vi "ProyectoFinalVI.vi"() -> ()   [LabVIEW 2025]
uses:
  <vilib>/httpClient/PUTBuffer.vi
  <vilib>/httpClient/LabVIEWHTTPClient.lvlib
panel:
  in  "Tab Control":T1(tab)
  out "Planta":dbl(knob)
  in  "OK Button":bool
  in  "Set-Point":dbl(knob) scale=0.0..360.0
  in  "KP":dbl
  out "error PUT":errorcluster
  out "headers PUT":string
  out "body PUT":string
  in  "KI":dbl
  in  "KD":dbl
  in  "Dt":dbl
  out "SET-POINT":dbl
  out "KP":dbl
  out "KI":dbl
  out "KD":dbl
  out "Dt":dbl
  out "POS":dbl
  out "error GET":errorcluster
  out "headers GET":string
  out "body GET":string
  out "Boolean 2":bool
  out "Boolean":bool
  out "Secuencia":string
  out "Aceptar":bool
  out "error GET 2":errorcluster
  out "body GET 2":string
  out "headers GET 2":string
  out "error PUT 2":errorcluster
  out "body PUT 2":string
  out "headers PUT 2":string
  in  "Secuencia 2":string
  in  "Aceptar 2":bool
  in  "OK Button 2":bool
  out "Tank":dbl(slide) scale=0.0..100.0
  out "KP 2":dbl
  out "KI 2":dbl
  out "RPM":dbl
  out "error GET 3":errorcluster
  out "body GET 3":string
  out "headers GET 3":string
  out "error PUT 3":errorcluster
  out "body PUT 3":string
  out "headers PUT 3":string
  in  "OK Button 3":bool
  in  "KP 3":dbl
  in  "KI 3":dbl
  in  "RPM 2":dbl
  out "Thermometer":dbl(slide) scale=0.0..100.0
  out "K":dbl
  out "Ki":dbl
  out "Kd":dbl
  out "SetPoint":dbl
  out "Temp":dbl
  out "error GET 4":errorcluster
  out "body GET 4":string
  out "headers GET 4":string
  out "error PUT 4":errorcluster
  out "body PUT 4":string
  out "headers PUT 4":string
  in  "OK Button 4":bool
  in  "K 2":dbl
  in  "Ki 2":dbl
  in  "Kd 2":dbl
  in  "SetPoint 2":dbl
  in  "Temp 2":dbl
  out "KP 4":dbl
  out "KI 4":dbl
  out "RPM 3":dbl
  in  "KP 5":dbl
  in  "KI 5":dbl
  in  "RPM 4":dbl
  in  "OK Button 5":bool
  out "error GET 5":errorcluster
  out "body GET 5":string
  out "headers GET 5":string
  out "error PUT 5":errorcluster
  out "body PUT 5":string
  out "headers PUT 5":string
  out "K 3":dbl
  out "Ki 3":dbl
  out "Kd 3":dbl
  out "sp":dbl
  in  "K 4":dbl
  in  "Ki 4":dbl
  in  "Kd 4":dbl
  in  "sp 2":dbl
  in  "OK Button 6":bool
  out "error GET 6":errorcluster
  out "body GET 6":string
  out "headers GET 6":string
  out "error PUT 6":errorcluster
  out "body PUT 6":string
  out "headers PUT 6":string
  out "error GET 7":errorcluster
  out "body GET 7":string
  out "headers GET 7":string
  out "error PUT 7":errorcluster
  out "body PUT 7":string
  out "headers PUT 7":string
  out "KP 6":dbl
  out "KI 6":dbl
  out "RPM 5":dbl
  in  "KP 7":dbl
  in  "KI 7":dbl
  in  "RPM 6":dbl
  in  "OK Button 7":bool
  in  "stop":bool
  # "Instituto Politécnico Nacional"
  # "Unidad Profesional Interdisciplinaria de Ingeniería Campus Zacatecas"
  # "Instrumentación Virtual Aplicada"
  # "Current Data"
  # "Send Data"
  # "Current Data"
  # "Send Data"
  # "Current Data"
  # "Send Data"
  # "Current Data"
  # "Send Data"
  # "Current Data"
  # "Send Data"
  # "Current Data"
  # "Send Data"
  # "Current Data"
  # "Current Data"
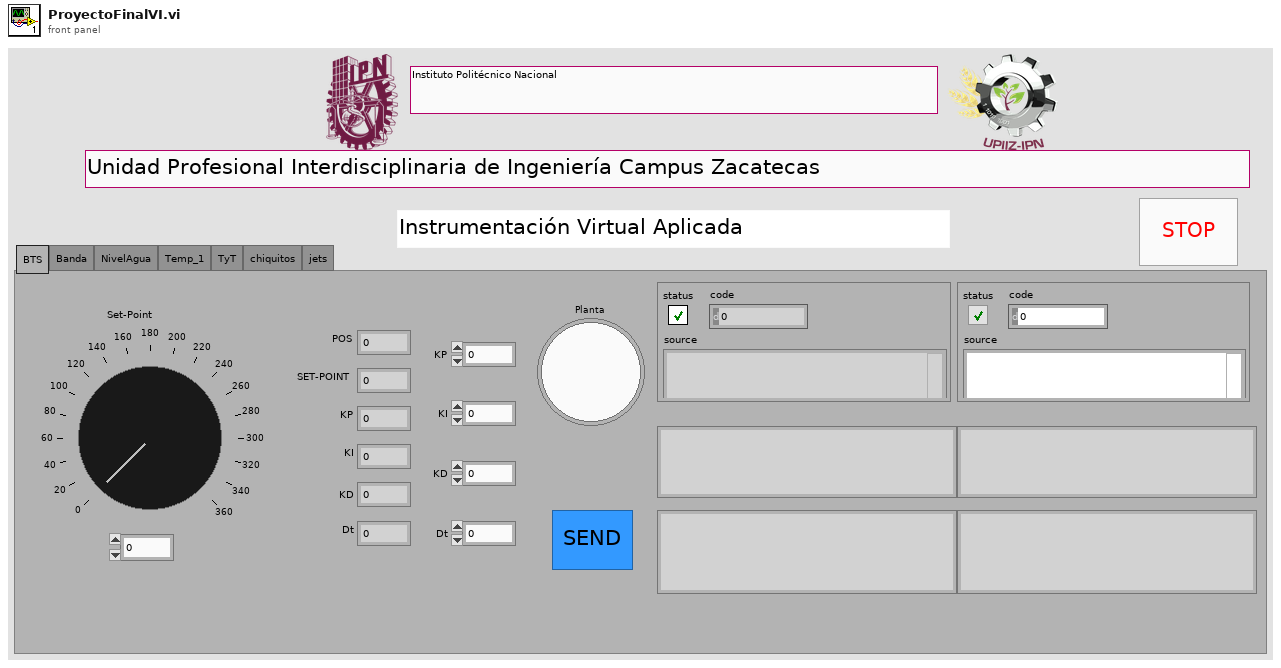
[diagram p1: front panel]
types:
  T1 = enum32{"BTS", "Banda", "NivelAgua", "Temp_1", "TyT", "chiquitos", "jets"}
  T2 = cluster{"Sensor":dbl, "Set-Point":dbl, "kp":dbl, "ki":dbl, "kd":dbl, "dt":dbl}
  T3 = cluster{"Set-Point":dbl, "kp":dbl, "ki":dbl, "kd":dbl, "dt":dbl, "Sensor":dbl}
  T4 = cluster{"K":dbl, "Ki":dbl, "Kd":dbl, "SetPoint":dbl, "Temp":dbl}
  T5 = cluster{"Kd":dbl, "Ki":dbl, "SetPoint":dbl, "Temp":dbl, "K":dbl}
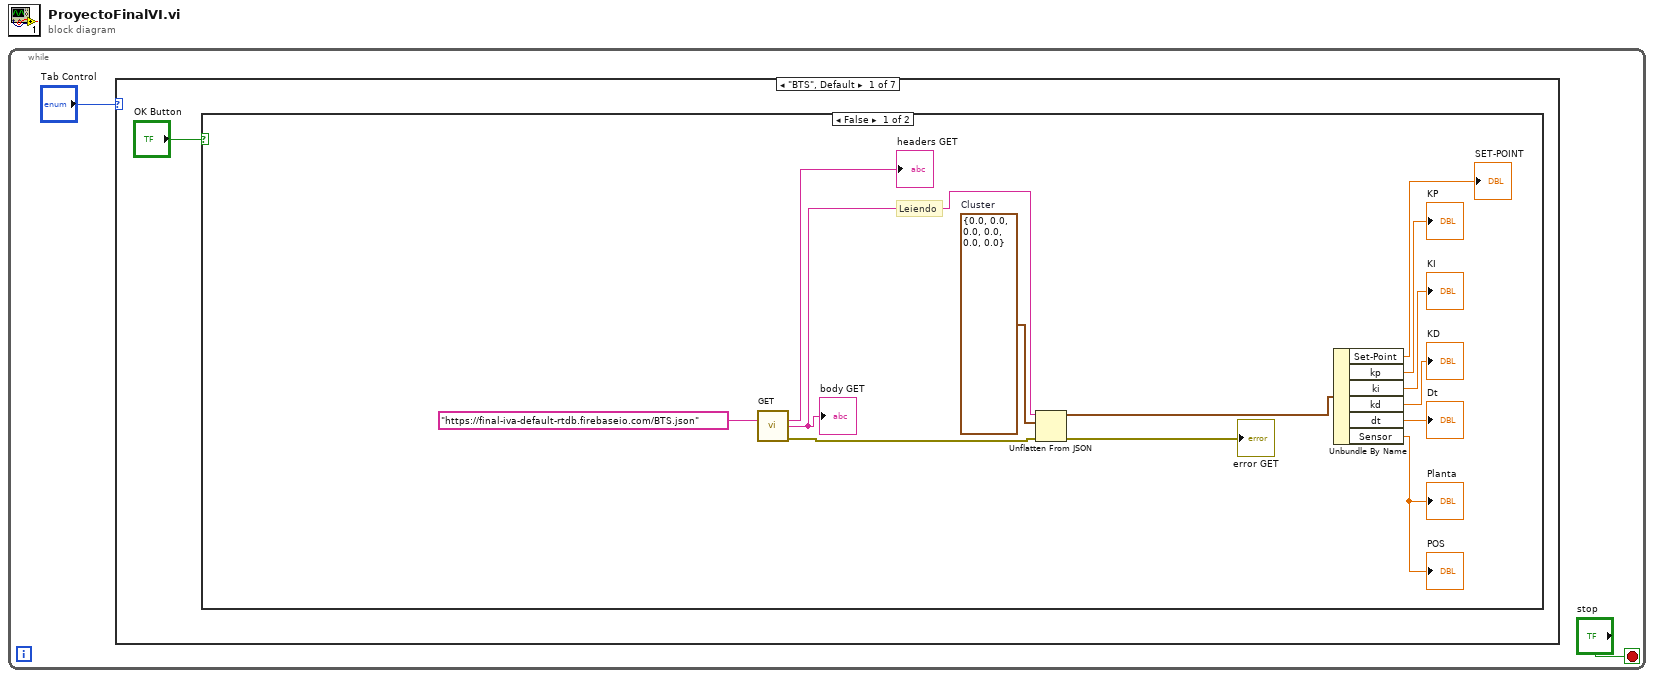
[diagram p0: block diagram]
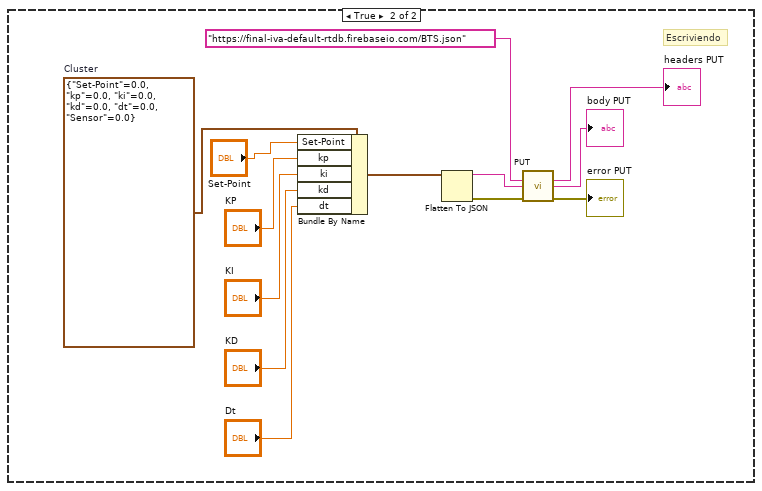
[diagram p2: hidden frame]
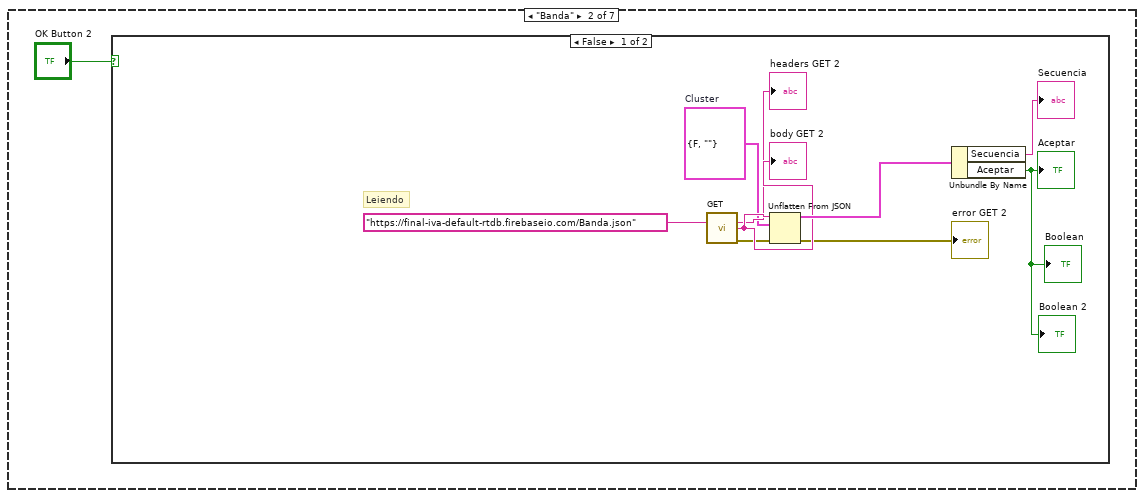
[diagram p3: hidden frame]
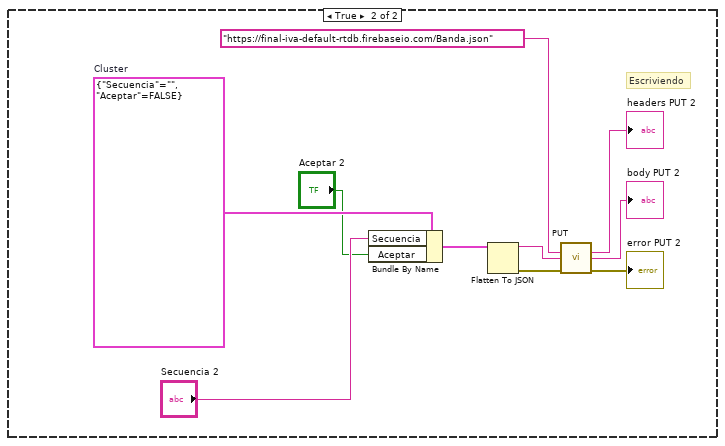
[diagram p4: hidden frame]
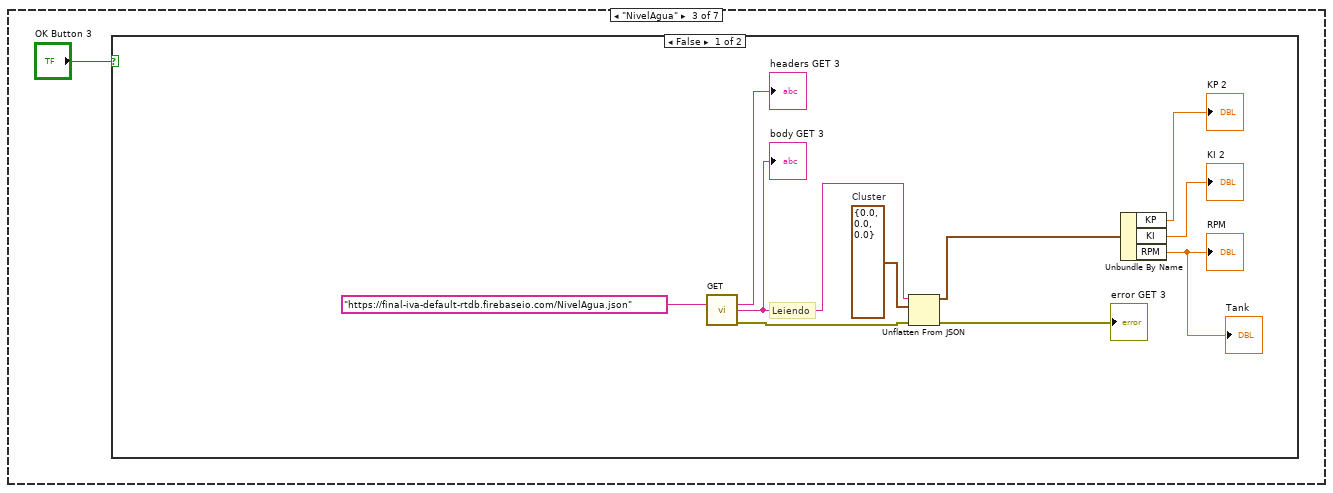
[diagram p5: hidden frame]
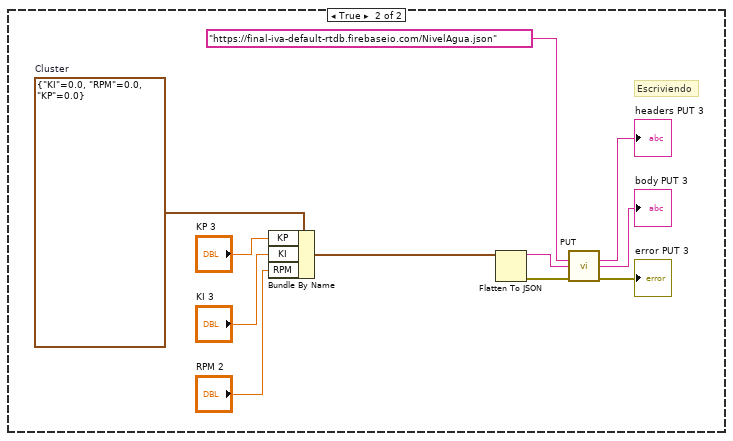
[diagram p6: hidden frame]
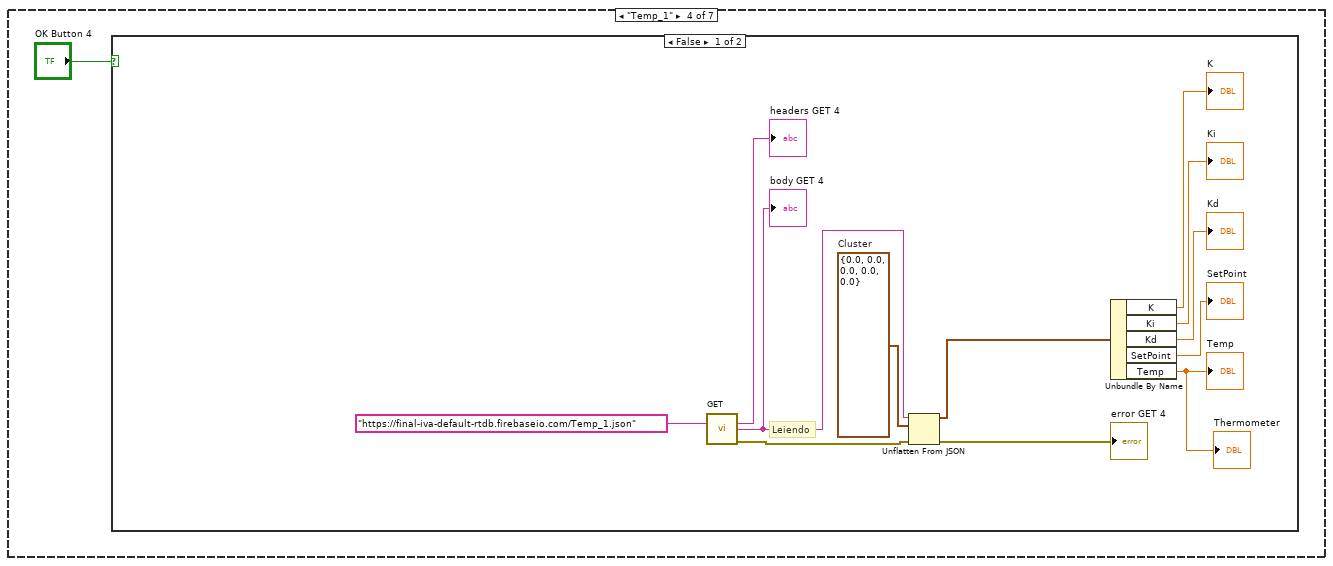
[diagram p7: hidden frame]
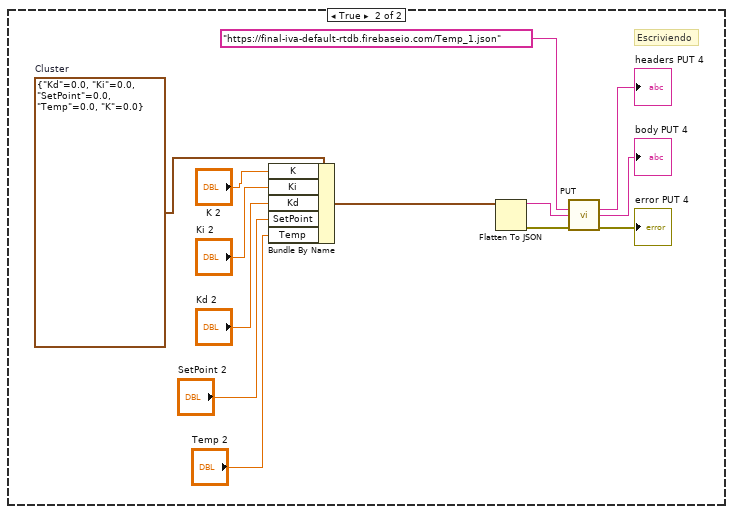
[diagram p8: hidden frame]
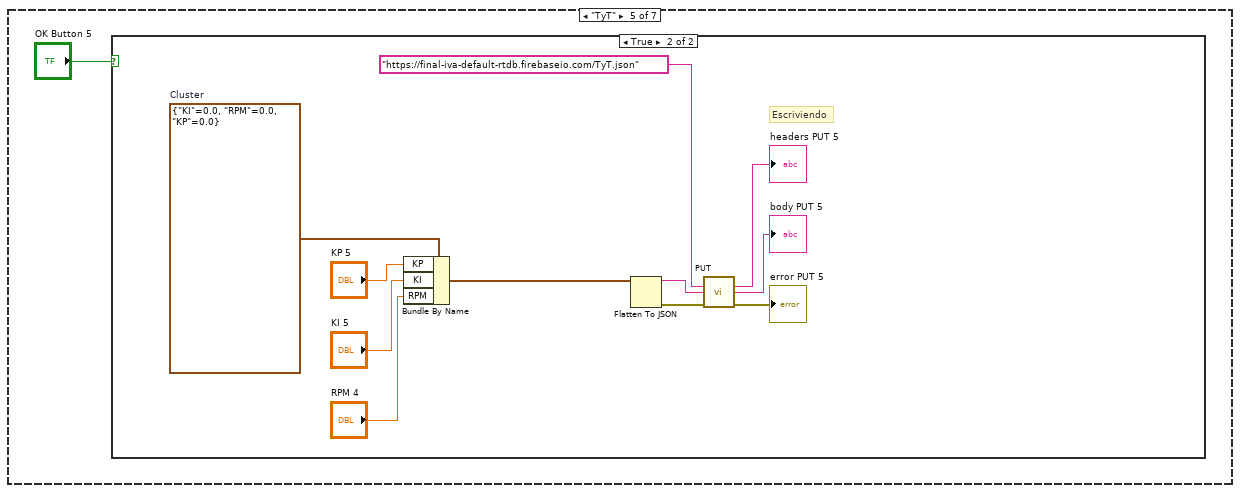
[diagram p9: hidden frame]
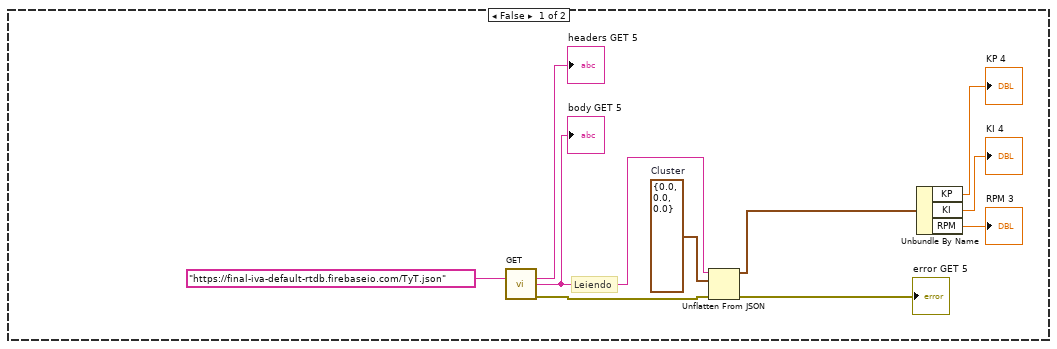
[diagram p10: hidden frame]
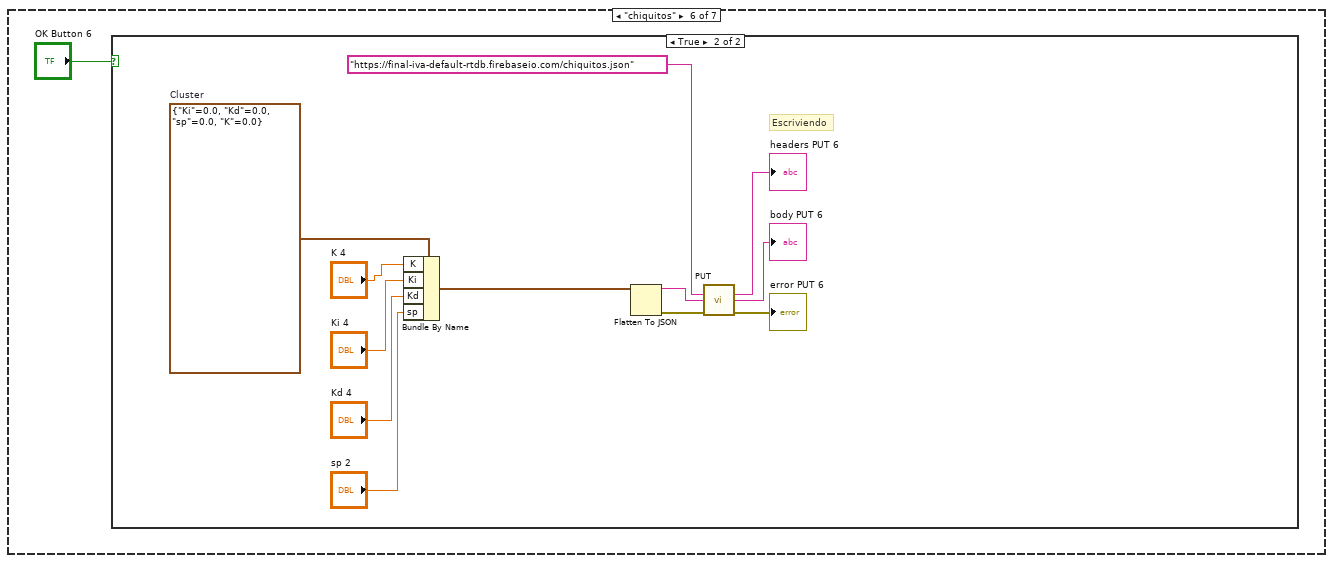
[diagram p11: hidden frame]
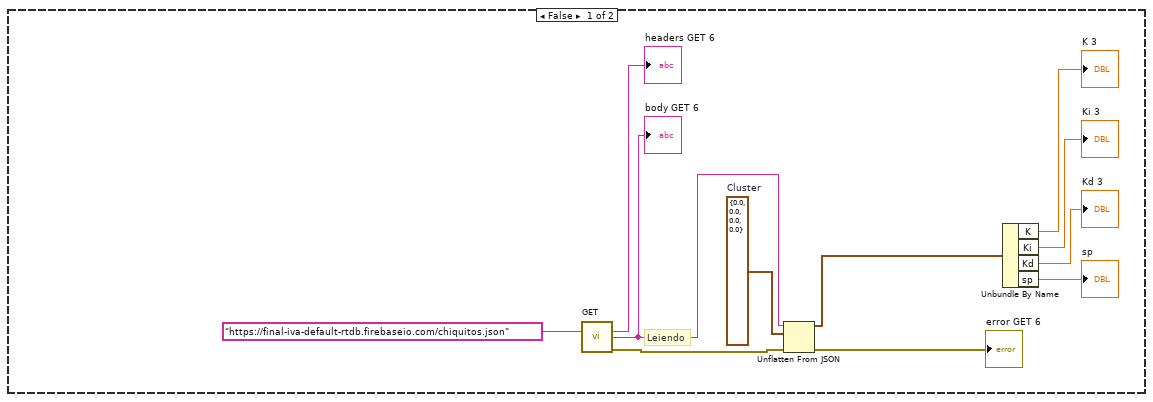
[diagram p12: hidden frame]
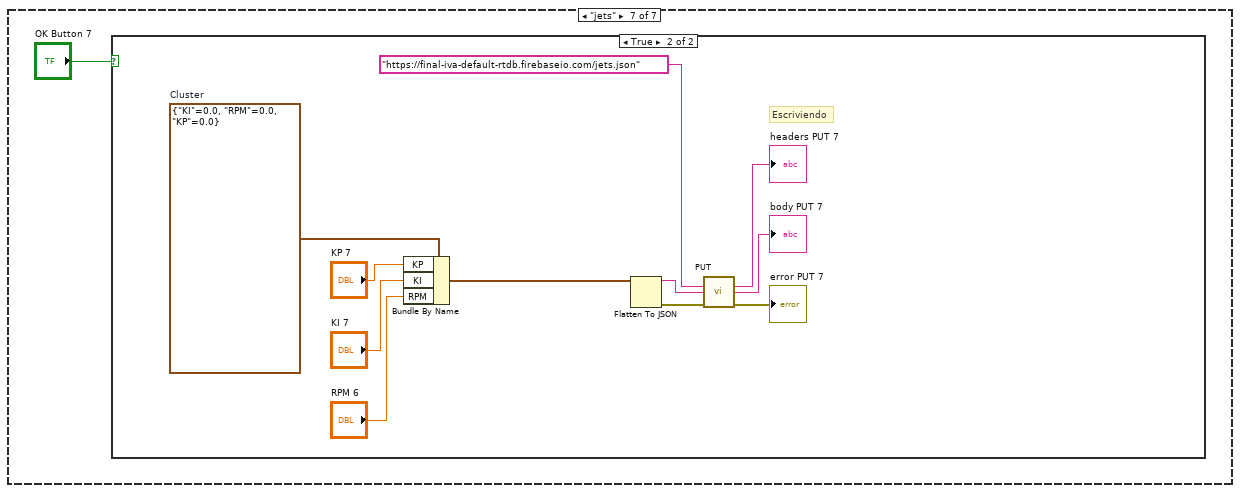
[diagram p13: hidden frame]
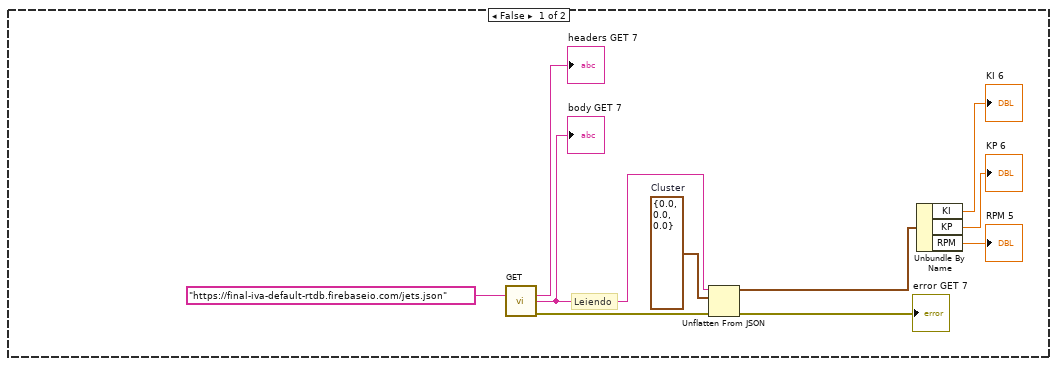
[diagram p14: hidden frame]
diagram:
  n1 = while {
    stop <- "stop" stop-if-true
    n2 = case shown="\"BTS\", Default" "Tab Control" {
      frame "BTS", Default {
        n3 = case shown="False" "OK Button" {
          frame False {
            w10 = T2 {"Sensor"=0.0, "Set-Point"=0.0, "kp"=0.0, "ki"=0.0, "kd"=0.0, "dt"=0.0}  # Cluster
            # "Leiendo"
            n4 = call <vilib>:"GET.vi"("url"="https://final-iva-default-rtdb.firebaseio.com/BTS.json") -> ("headers"=→"headers GET":string, "body"=w15:string, "error out"=w12:errorcluster)  [unwired: 11 in, 1 out]
            "body GET" <- w15
            n5 = Unflatten From JSON(JSON string=w15, type and defaults=w10, error in (no error)=w12) -> (value=w16:T2, error out=→"error GET":errorcluster)  [unwired: 4 in]
            n6 = Unbundle By Name(w16) -> ("Set-Point"=→"SET-POINT":dbl, "kp"=→"KP":dbl, "ki"=→"KI":dbl, "kd"=→"KD":dbl, "dt"=→"Dt":dbl, "Sensor"=→"POS" →"Planta":dbl)
          }
          frame True {
            w23 = T3 {"Set-Point"=0.0, "kp"=0.0, "ki"=0.0, "kd"=0.0, "dt"=0.0, "Sensor"=0.0}  # Cluster
            # "Escriviendo"
            n7 = Bundle By Name "Bundle By Name"(cluster=w23, "Set-Point"="Set-Point", "kp"="KP", "ki"="KI", "kd"="KD", "dt"="Dt") -> (w29:T3)
            n8 = Flatten To JSON(anything=w29) -> (JSON string=w26:string, 11:w22:errorcluster)  [unwired: 2 in]
            n9 = call-poly <vilib>:"PUT.vi"("url"="https://final-iva-default-rtdb.firebaseio.com/BTS.json", "buffer"=w26, "error in (no error)"=w22) -> ("headers"=→"headers PUT":string, "body"=→"body PUT":string, "error out"=→"error PUT":errorcluster)  [unwired: 9 in, 1 out]
          }
        }
      }
      frame "Banda" {
        n10 = case shown="False" "OK Button 2" {
          frame False {
            w33 = cluster{"Aceptar":bool, "Secuencia":string} {"Aceptar"=FALSE, "Secuencia"=""}  # Cluster
            # "Leiendo"
            n11 = call <vilib>:"GET.vi"("url"="https://final-iva-default-rtdb.firebaseio.com/Banda.json") -> ("headers"=→"headers GET 2":string, "body"=w38:string, "error out"=w35:errorcluster)  [unwired: 11 in, 1 out]
            "body GET 2" <- w38
            n12 = Unflatten From JSON(JSON string=w38, type and defaults=w33, error in (no error)=w35) -> (value=w39:cluster{"Aceptar":bool, "Secuencia":string}, error out=→"error GET 2":errorcluster)  [unwired: 4 in]
            n13 = Unbundle By Name(w39) -> ("Secuencia"=→"Secuencia":string, "Aceptar"=→"Aceptar" →"Boolean" →"Boolean 2":bool)
          }
          frame True {
            w43 = cluster{"Secuencia":string, "Aceptar":bool} {"Secuencia"="", "Aceptar"=FALSE}  # Cluster
            # "Escriviendo"
            n14 = Bundle By Name "Bundle By Name"(cluster=w43, "Secuencia"="Secuencia 2", "Aceptar"="Aceptar 2") -> (w49:cluster{"Secuencia":string, "Aceptar":bool})
            n15 = Flatten To JSON(anything=w49) -> (JSON string=w46:string, 11:w42:errorcluster)  [unwired: 2 in]
            n16 = call-poly <vilib>:"PUT.vi"("url"="https://final-iva-default-rtdb.firebaseio.com/Banda.json", "buffer"=w46, "error in (no error)"=w42) -> ("headers"=→"headers PUT 2":string, "body"=→"body PUT 2":string, "error out"=→"error PUT 2":errorcluster)  [unwired: 9 in, 1 out]
          }
        }
      }
      frame "NivelAgua" {
        n17 = case shown="False" "OK Button 3" {
          frame False {
            w54 = cluster{"KP":dbl, "KI":dbl, "RPM":dbl} {"KP"=0.0, "KI"=0.0, "RPM"=0.0}  # Cluster
            # "Leiendo"
            n18 = call <vilib>:"GET.vi"("url"="https://final-iva-default-rtdb.firebaseio.com/NivelAgua.json") -> ("headers"=→"headers GET 3":string, "body"=w59:string, "error out"=w56:errorcluster)  [unwired: 11 in, 1 out]
            "body GET 3" <- w59
            n19 = Unflatten From JSON(JSON string=w59, type and defaults=w54, error in (no error)=w56) -> (value=w60:cluster{"KP":dbl, "KI":dbl, "RPM":dbl}, error out=→"error GET 3":errorcluster)  [unwired: 4 in]
            n20 = Unbundle By Name(w60) -> ("KP"=→"KP 2":dbl, "KI"=→"KI 2":dbl, "RPM"=→"RPM" →"Tank":dbl)
          }
          frame True {
            w65 = cluster{"KI":dbl, "RPM":dbl, "KP":dbl} {"KI"=0.0, "RPM"=0.0, "KP"=0.0}  # Cluster
            # "Escriviendo"
            n21 = Bundle By Name "Bundle By Name"(cluster=w65, "KP"="KP 3", "KI"="KI 3", "RPM"="RPM 2") -> (w71:cluster{"KI":dbl, "RPM":dbl, "KP":dbl})
            n22 = Flatten To JSON(anything=w71) -> (JSON string=w68:string, 11:w64:errorcluster)  [unwired: 2 in]
            n23 = call-poly <vilib>:"PUT.vi"("url"="https://final-iva-default-rtdb.firebaseio.com/NivelAgua.json", "buffer"=w68, "error in (no error)"=w64) -> ("headers"=→"headers PUT 3":string, "body"=→"body PUT 3":string, "error out"=→"error PUT 3":errorcluster)  [unwired: 9 in, 1 out]
          }
        }
      }
      frame "Temp_1" {
        n24 = case shown="False" "OK Button 4" {
          frame False {
            w78 = T4 {"K"=0.0, "Ki"=0.0, "Kd"=0.0, "SetPoint"=0.0, "Temp"=0.0}  # Cluster
            # "Leiendo"
            n25 = call <vilib>:"GET.vi"("url"="https://final-iva-default-rtdb.firebaseio.com/Temp_1.json") -> ("headers"=→"headers GET 4":string, "body"=w83:string, "error out"=w80:errorcluster)  [unwired: 11 in, 1 out]
            "body GET 4" <- w83
            n26 = Unflatten From JSON(JSON string=w83, type and defaults=w78, error in (no error)=w80) -> (value=w84:T4, error out=→"error GET 4":errorcluster)  [unwired: 4 in]
            n27 = Unbundle By Name(w84) -> ("K"=→"K":dbl, "Ki"=→"Ki":dbl, "Kd"=→"Kd":dbl, "SetPoint"=→"SetPoint":dbl, "Temp"=→"Temp" →"Thermometer":dbl)
          }
          frame True {
            w91 = T5 {"Kd"=0.0, "Ki"=0.0, "SetPoint"=0.0, "Temp"=0.0, "K"=0.0}  # Cluster
            # "Escriviendo"
            n28 = Bundle By Name "Bundle By Name"(cluster=w91, "K"="K 2", "Ki"="Ki 2", "Kd"="Kd 2", "SetPoint"="SetPoint 2", "Temp"="Temp 2") -> (w97:T5)
            n29 = Flatten To JSON(anything=w97) -> (JSON string=w94:string, 11:w90:errorcluster)  [unwired: 2 in]
            n30 = call-poly <vilib>:"PUT.vi"("url"="https://final-iva-default-rtdb.firebaseio.com/Temp_1.json", "buffer"=w94, "error in (no error)"=w90) -> ("headers"=→"headers PUT 4":string, "body"=→"body PUT 4":string, "error out"=→"error PUT 4":errorcluster)  [unwired: 9 in, 1 out]
          }
        }
      }
      frame "TyT" {
        n31 = case shown="True" "OK Button 5" {
          frame False {
            w102 = cluster{"KP":dbl, "KI":dbl, "RPM":dbl} {"KP"=0.0, "KI"=0.0, "RPM"=0.0}  # Cluster
            # "Leiendo"
            n32 = call <vilib>:"GET.vi"("url"="https://final-iva-default-rtdb.firebaseio.com/TyT.json") -> ("headers"=→"headers GET 5":string, "body"=w107:string, "error out"=w104:errorcluster)  [unwired: 11 in, 1 out]
            "body GET 5" <- w107
            n33 = Unflatten From JSON(JSON string=w107, type and defaults=w102, error in (no error)=w104) -> (value=w108:cluster{"KP":dbl, "KI":dbl, "RPM":dbl}, error out=→"error GET 5":errorcluster)  [unwired: 4 in]
            n34 = Unbundle By Name(w108) -> ("KP"=→"KP 4":dbl, "KI"=→"KI 4":dbl, "RPM"=→"RPM 3":dbl)
          }
          frame True {
            w113 = cluster{"KI":dbl, "RPM":dbl, "KP":dbl} {"KI"=0.0, "RPM"=0.0, "KP"=0.0}  # Cluster
            # "Escriviendo"
            n35 = Bundle By Name "Bundle By Name"(cluster=w113, "KP"="KP 5", "KI"="KI 5", "RPM"="RPM 4") -> (w119:cluster{"KI":dbl, "RPM":dbl, "KP":dbl})
            n36 = Flatten To JSON(anything=w119) -> (JSON string=w116:string, 11:w112:errorcluster)  [unwired: 2 in]
            n37 = call-poly <vilib>:"PUT.vi"("url"="https://final-iva-default-rtdb.firebaseio.com/TyT.json", "buffer"=w116, "error in (no error)"=w112) -> ("headers"=→"headers PUT 5":string, "body"=→"body PUT 5":string, "error out"=→"error PUT 5":errorcluster)  [unwired: 9 in, 1 out]
          }
        }
      }
      frame "chiquitos" {
        n38 = case shown="True" "OK Button 6" {
          frame False {
            w125 = cluster{"K":dbl, "Ki":dbl, "Kd":dbl, "sp":dbl} {"K"=0.0, "Ki"=0.0, "Kd"=0.0, "sp"=0.0}  # Cluster
            # "Leiendo"
            n39 = call <vilib>:"GET.vi"("url"="https://final-iva-default-rtdb.firebaseio.com/chiquitos.json") -> ("headers"=→"headers GET 6":string, "body"=w130:string, "error out"=w127:errorcluster)  [unwired: 11 in, 1 out]
            "body GET 6" <- w130
            n40 = Unflatten From JSON(JSON string=w130, type and defaults=w125, error in (no error)=w127) -> (value=w131:cluster{"K":dbl, "Ki":dbl, "Kd":dbl, "sp":dbl}, error out=→"error GET 6":errorcluster)  [unwired: 4 in]
            n41 = Unbundle By Name(w131) -> ("K"=→"K 3":dbl, "Ki"=→"Ki 3":dbl, "Kd"=→"Kd 3":dbl, "sp"=→"sp":dbl)
          }
          frame True {
            w137 = cluster{"Ki":dbl, "Kd":dbl, "sp":dbl, "K":dbl} {"Ki"=0.0, "Kd"=0.0, "sp"=0.0, "K"=0.0}  # Cluster
            # "Escriviendo"
            n42 = Bundle By Name "Bundle By Name"(cluster=w137, "K"="K 4", "Ki"="Ki 4", "Kd"="Kd 4", "sp"="sp 2") -> (w143:cluster{"Ki":dbl, "Kd":dbl, "sp":dbl, "K":dbl})
            n43 = Flatten To JSON(anything=w143) -> (JSON string=w140:string, 11:w136:errorcluster)  [unwired: 2 in]
            n44 = call-poly <vilib>:"PUT.vi"("url"="https://final-iva-default-rtdb.firebaseio.com/chiquitos.json", "buffer"=w140, "error in (no error)"=w136) -> ("headers"=→"headers PUT 6":string, "body"=→"body PUT 6":string, "error out"=→"error PUT 6":errorcluster)  [unwired: 9 in, 1 out]
          }
        }
      }
      frame "jets" {
        n45 = case shown="True" "OK Button 7" {
          frame False {
            w148 = cluster{"KI":dbl, "KP":dbl, "RPM":dbl} {"KI"=0.0, "KP"=0.0, "RPM"=0.0}  # Cluster
            # "Leiendo"
            n46 = call <vilib>:"GET.vi"("url"="https://final-iva-default-rtdb.firebaseio.com/jets.json") -> ("headers"=→"headers GET 7":string, "body"=w153:string, "error out"=w150:errorcluster)  [unwired: 11 in, 1 out]
            "body GET 7" <- w153
            n47 = Unflatten From JSON(JSON string=w153, type and defaults=w148, error in (no error)=w150) -> (value=w154:cluster{"KI":dbl, "KP":dbl, "RPM":dbl}, error out=→"error GET 7":errorcluster)  [unwired: 4 in]
            n48 = Unbundle By Name(w154) -> ("KI"=→"KI 6":dbl, "KP"=→"KP 6":dbl, "RPM"=→"RPM 5":dbl)
          }
          frame True {
            w159 = cluster{"KI":dbl, "RPM":dbl, "KP":dbl} {"KI"=0.0, "RPM"=0.0, "KP"=0.0}  # Cluster
            # "Escriviendo"
            n49 = Bundle By Name "Bundle By Name"(cluster=w159, "KP"="KP 7", "KI"="KI 7", "RPM"="RPM 6") -> (w165:cluster{"KI":dbl, "RPM":dbl, "KP":dbl})
            n50 = Flatten To JSON(anything=w165) -> (JSON string=w162:string, 11:w158:errorcluster)  [unwired: 2 in]
            n51 = call-poly <vilib>:"PUT.vi"("url"="https://final-iva-default-rtdb.firebaseio.com/jets.json", "buffer"=w162, "error in (no error)"=w158) -> ("headers"=→"headers PUT 7":string, "body"=→"body PUT 7":string, "error out"=→"error PUT 7":errorcluster)  [unwired: 9 in, 1 out]
          }
        }
      }
    }
  }
